vi "Trial.vi"() -> ()   [LabVIEW 2024]
uses:
  <vilib>/Utility/NIReport.llb/Report Type.ctl
  <vilib>/Utility/NIReport.llb/Append Text Table to Report (wrap).vi
  <vilib>/Utility/NIReport.llb/NI_report.lvclass
  <vilib>/Utility/NIReport.llb/NI_ReportGenerationCore.lvlib
  <vilib>/Utility/NIReport.llb/Excel/NI_Excel.lvclass
panel:
  out "array":string[][](array[string])
  out "text":string
  out "filenames":string[](array[string])
  out "concatenated string":string
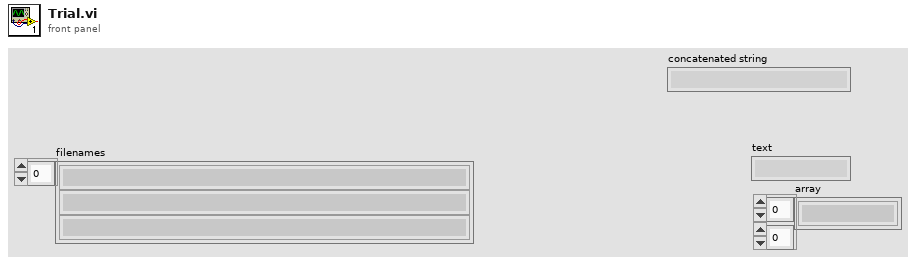
[diagram p1: front panel]
types:
  T1 = typedef "NI_ReportGenerationCore.lvlib/Report Type.ctl" = enum16{"HTML", "Word", "Excel"}
  T2 = enum16{"maximized", "minimized", "normal", "no change"}
  T3 = typedef "LVDateTimeRec.ctl" = cluster{"fractional second":dbl, "second":i32, "minute":i32, "hour":i32, "day of month":i32, "month":i32, "year":i32, "day of week":i32, "day of year":i32, "DST":i32}
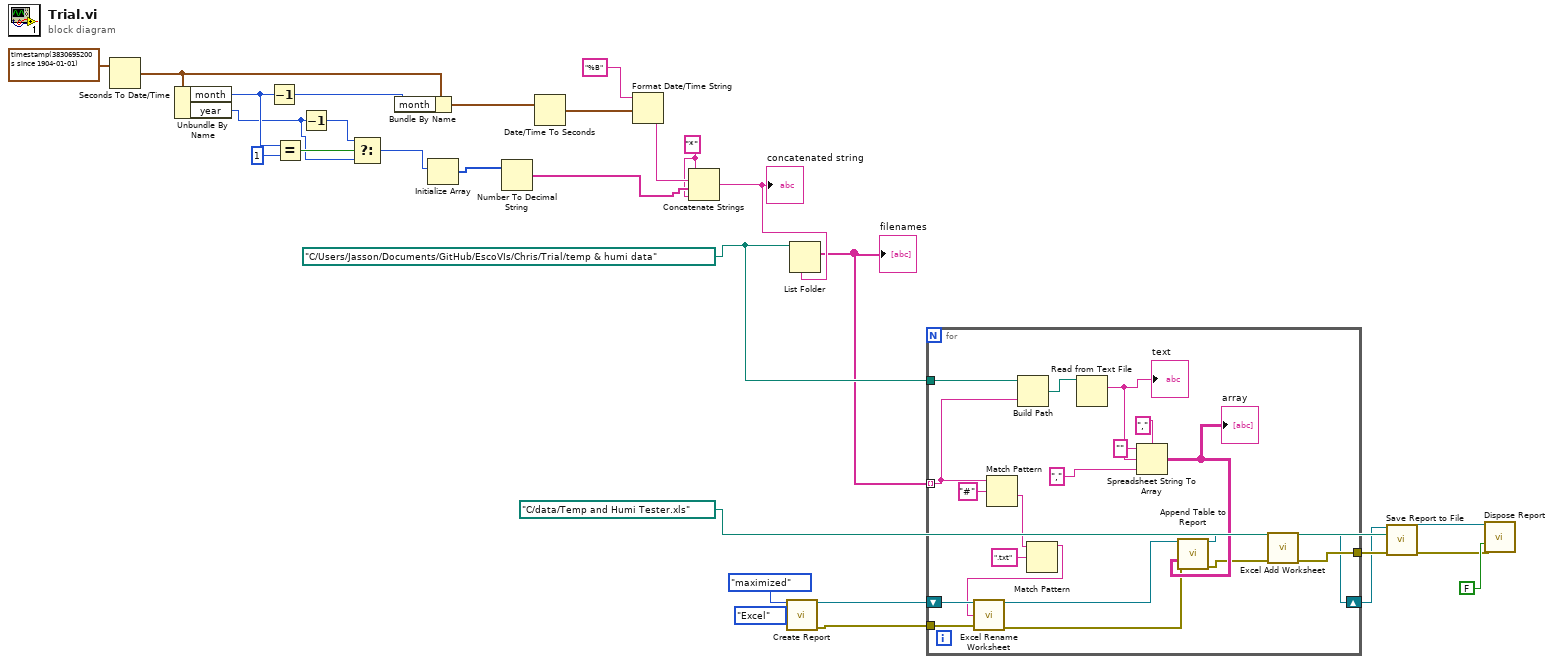
[diagram p0: block diagram]
diagram:
  w12 = path "C:/Users/Jasson/Documents/GitHub/EscoVIs/Chris/Trial/temp & humi data" ("path")
  w14 = "*" ("string")
  n1 = Seconds To Date/Time(time stamp (now)=timestamp(3830695200 s since 1904-01-01) ("time stamp")) -> (date time rec=w22:T3)  [unwired: 1 in]
  n2 = Unbundle By Name(w22) -> ("month"=w28:i32, "year"=w24:i32)
  n3 = Decrement(x=w28) -> (x-1=w23:i32)
  n4 = Equal?(x=w28, y=1) -> (x = y?=w26:bool)
  n5 = Decrement(x=w24) -> (x-1=w25:i32)
  n6 = Select(t=w25, s=w26, f=w24) -> (s? t:f=w18:i32)
  n7 = Bundle By Name(cluster=w22, "month"=w23) -> (w21:T3)
  n8 = Initialize Array(w18) -> (w17:i32[])  [unwired: 1 in]
  n9 = Number To Decimal String(number=w17) -> (decimal integer string=w16:string[])  [unwired: 1 in]
  n10 = Date/Time To Seconds(2:w21) -> (0:w20:timestamp)  [unwired: 1 in]
  n11 = Format Date/Time String(time format string (%c)="%B", seconds (now)=w20) -> (date/time string=w15:string)  [unwired: 1 in]
  n12 = Concatenate Strings(w14, w15, w16, w14) -> (w13:string)
  "concatenated string" <- w13
  n13 = call <vilib>:"Create Report.vi"("window state (normal)"=T2."maximized", "report type"=Report_Type."Excel") -> ("report out"=w8:refnum<class "NI_report.lvclass">, "error out"=w4:errorcluster)  [unwired: 12 in]
  n14 = List Folder(path=w12, pattern=w13) -> (filenames=w2:string[])  [unwired: 2 in, 3 out]
  "filenames" <- w2
  n15 = for {
    tunnel: w2 -> [w33] mode=indexing
    tunnel: w12 -> [w49]
    tunnel: w4 -> [w41]
    tunnel: [w36] -> w3
    shift-right: [w30] -> w1
    shift-left: w8 -> [w42]
    n16 = Match Pattern(string=w33, regular expression="#") -> (after substring=w31:string)  [unwired: 1 in, 3 out]
    n17 = Build Path(base path=w49, name or relative path=w33) -> (appended path=w48:path)
    n18 = Match Pattern(string=w31, regular expression=".txt") -> (before substring=w34:string)  [unwired: 1 in, 3 out]
    n19 = call <vilib>:"Excel Rename Worksheet.vi"("report in"=w42, "worksheet name (\"\")"=w34, "error in (no error)"=w41) -> ("report out"=w40:refnum<class "NI_report.lvclass">, "error out"=w39:errorcluster)  [unwired: 11 in]
    n20 = Read from Text File(file (use dialog)=w48) -> (text=w47:string)  [unwired: 3 in, 3 out]
    "text" <- w47
    n21 = Spreadsheet String To Array(delimiter (Tab)=",", format string="", spreadsheet string=w47, array type (2D Dbl)=",") -> (array=w43:string[][])
    "array" <- w43
    n22 = call-poly <vilib>:"Append Table to Report.vi"("report in"=w40, "text data"=w43, "error in (no error)"=w39) -> ("report out"=w38:refnum<class "NI_report.lvclass">, "error out"=w37:errorcluster)  [unwired: 9 in, 2 out]
    n23 = call <vilib>:"Excel Add Worksheet.vi"("report in"=w38, "error in (no error)"=w37) -> ("report out"=w30:refnum<class "NI_report.lvclass">, "error out"=w36:errorcluster)  [unwired: 12 in]
  }
  n24 = call-dynamic "Save Report to File.vi"("report in"=w1, "report file path"=path "C:/data/Temp and Humi Tester.xls", "error in (no error)"=w3) -> ("report out"=w5:refnum<class "NI_report.lvclass">, "error out"=w6:errorcluster)  [unwired: 11 in]
  n25 = call-dynamic "Dispose Report.vi"("report in"=w5, "save changes? (F)"=FALSE, "error in (no error)"=w6) -> ()  [unwired: 12 in, 1 out]
